vi "Read WorkTable.vi"(8 "error in":errorcluster, 11 "Gantry Class in":refnum<class "Gantry Class.lvclass">) -> (0 "error out":errorcluster, 2 "WorkTable Class.lvclass":refnum<class "WorkTable Class.lvclass">, 3 "Gantry Class out":refnum<class "Gantry Class.lvclass">)   [LabVIEW 2011, in "Gantry Class.lvclass"]
uses:
  Gantry Class.lvclass
  WorkTable Class/WorkTable Class.lvclass
  Gantry Class.lvclass/Gantry Class.ctl
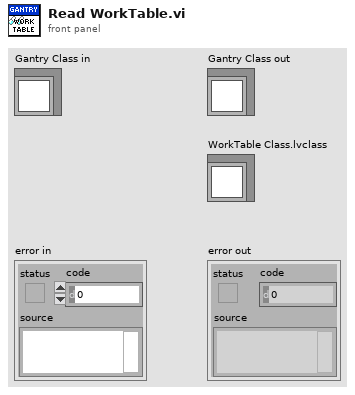
[diagram p1: front panel]
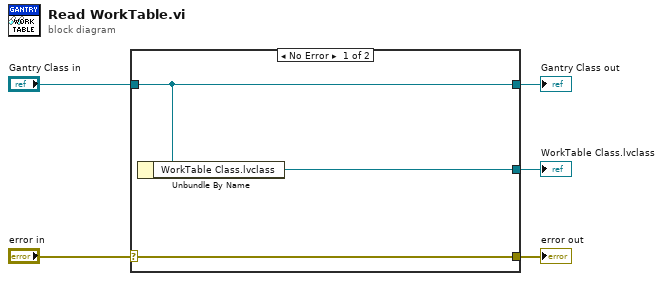
[diagram p0: block diagram]
diagram:
  n1 = case shown="No Error" "error in" {
    selector: "error in" -> [w8 w9]
    tunnel: [w8 w9] -> w4
    tunnel: [w7 w10] -> w2
    tunnel: "Gantry Class in" -> [w7 w10]
    tunnel: [w6 _] -> w1
    frame No Error {
      n2 = Unbundle By Name(w7) -> ("WorkTable Class.lvclass"=w6:refnum<class "WorkTable Class.lvclass">)
    }
    frame Error {
    }
  }
  "error out" <- w4
  "Gantry Class out" <- w2
  "WorkTable Class.lvclass" <- w1
